vi "FTDI_Status_Explanation.vi"(1 "FT_Status":u32) -> (0 "Status String":string)   [LabVIEW 2011]
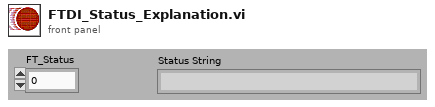
[diagram p1: front panel]
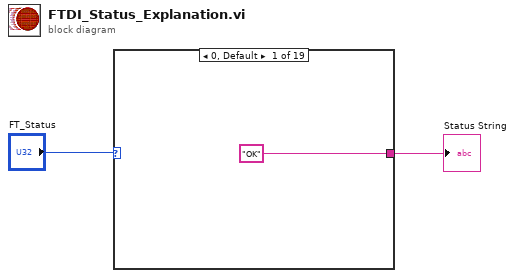
[diagram p0: block diagram]
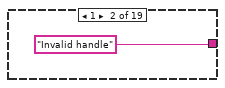
[diagram p2: hidden frame]
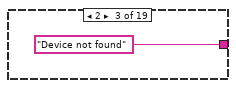
[diagram p3: hidden frame]
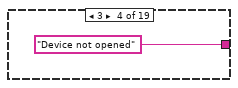
[diagram p4: hidden frame]
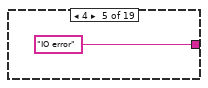
[diagram p5: hidden frame]
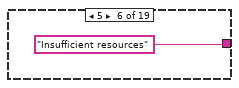
[diagram p6: hidden frame]
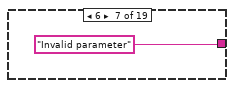
[diagram p7: hidden frame]
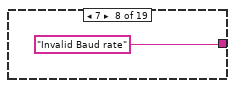
[diagram p8: hidden frame]
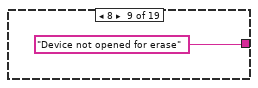
[diagram p9: hidden frame]
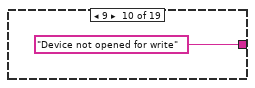
[diagram p10: hidden frame]
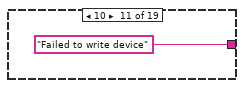
[diagram p11: hidden frame]
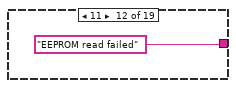
[diagram p12: hidden frame]
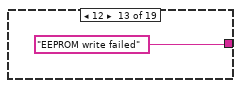
[diagram p13: hidden frame]
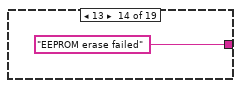
[diagram p14: hidden frame]
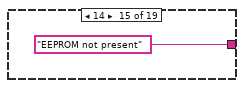
[diagram p15: hidden frame]
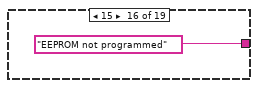
[diagram p16: hidden frame]
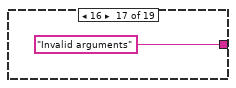
[diagram p17: hidden frame]
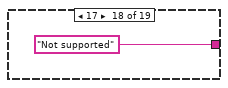
[diagram p18: hidden frame]
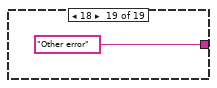
[diagram p19: hidden frame]
diagram:
  n1 = case shown="0, Default" "FT_Status" {
    tunnel: ["OK" "Invalid handle" "Device not found" "Device not opened" "IO error" "Insufficient resources" "Invalid parameter" "Invalid Baud rate" "Device not opened for erase" "Device not opened for write" "Failed to write device" "EEPROM read failed" "EEPROM write failed" "EEPROM erase failed" "EEPROM not present" "EEPROM not programmed" "Invalid arguments" "Not supported" "Other error"] -> w1
    frame 0, Default {
    }
    frame 1 {
    }
    frame 2 {
    }
    frame 3 {
    }
    frame 4 {
    }
    frame 5 {
    }
    frame 6 {
    }
    frame 7 {
    }
    frame 8 {
    }
    frame 9 {
    }
    frame 10 {
    }
    frame 11 {
    }
    frame 12 {
    }
    frame 13 {
    }
    frame 14 {
    }
    frame 15 {
    }
    frame 16 {
    }
    frame 17 {
    }
    frame 18 {
    }
  }
  "Status String" <- w1
